vi "runScript.vi"(6 "timeStamp":string, 8 "error in (no error)":errorcluster, 9 "Path":path, 10 "CompiledScript":T1, 11 "BECHWCBasic in":refnum<class "BECHWCBasic.lvclass">) -> (0 "error out":errorcluster, 3 "BECHWCBasic out":refnum<class "BECHWCBasic.lvclass">)   [LabVIEW 2011, in "Hardware.lvlib" / "HWControllers.lvlib" / "BECHWCBasic.lvclass"]
uses:
  BECHWCBasic.lvclass
  Tools/SettingsProcessors/ScriptListCompiler/ScriptListCompiler.lvclass
  Channels/VoltOutput/AnalogOutput.lvclass
  Channels/Digital/DigitalOutput.lvclass
  Channels/DDSOutput/Generic/DDSOutput.lvclass
  HWController.lvclass
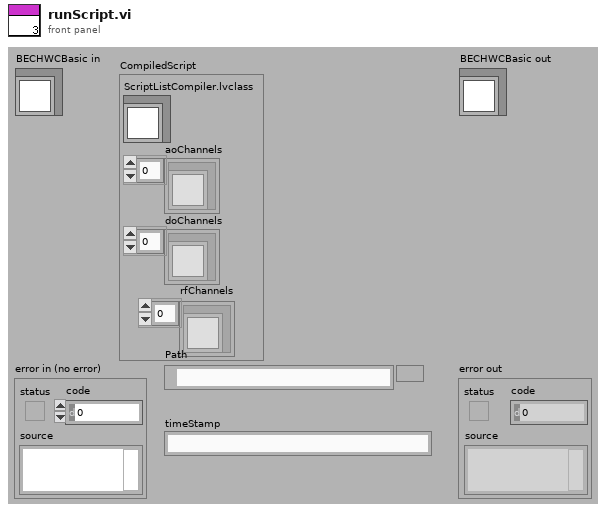
[diagram p1: front panel]
types:
  T1 = cluster{"ScriptListCompiler.lvclass":refnum<class "ScriptListCompiler.lvclass">, "aoChannels":refnum<class "AnalogOutput.lvclass">[], "doChannels":refnum<class "DigitalOutput.lvclass">[], "rfChannels":refnum<class "DDSOutput.lvclass">[]}
  T2 = enum16{"Ready", "Compiling", "Configured", "Running", "Stopping", "Unresolved Error"}
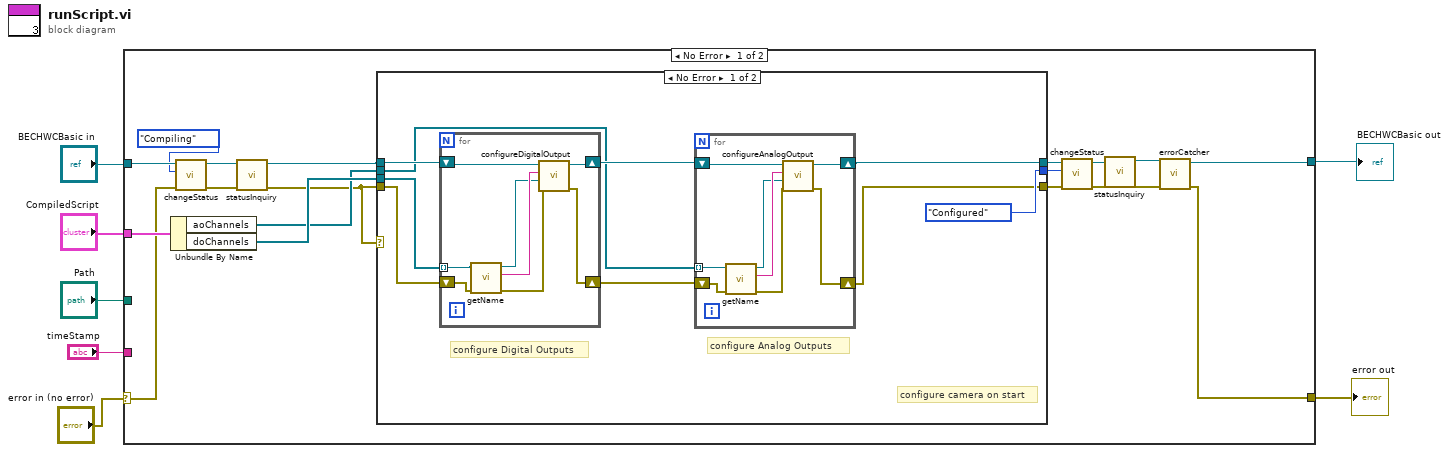
[diagram p0: block diagram]
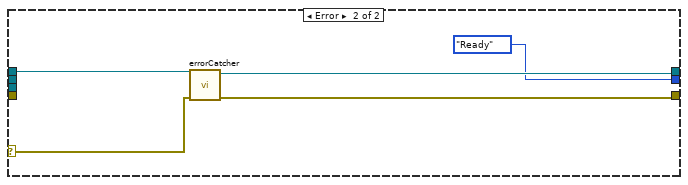
[diagram p2: hidden frame]
diagram:
  n1 = case shown="No Error" "error in (no error)" {
    selector: "error in (no error)" -> [w12 w57]
    tunnel: "BECHWCBasic in" -> [w20 w58]
    tunnel: [w9 w58] -> w5
    tunnel: [w8 w57] -> w4
    tunnel: "CompiledScript" -> [w17 _]
    tunnel: "timeStamp" -> [_ _]
    tunnel: "Path" -> [_ _]
    frame No Error {
      n2 = Unbundle By Name(w17) -> ("aoChannels"=w15:refnum<class "AnalogOutput.lvclass">[], "doChannels"=w16:refnum<class "DigitalOutput.lvclass">[])
      n3 = call "changeStatus.vi"("error in (no error)"=w12, "status"=T2."Compiling", "HWController in"=w20) -> ("error out"=w22:errorcluster, "HWController out"=w21:refnum<class "BECHWCBasic.lvclass">)  [unwired: 7 in]
      n4 = call-dynamic "statusInquiry.vi"("error in (no error)"=w22, "HWController in"=w21) -> ("error out"=w13:errorcluster, "HWController out"=w14:refnum<class "BECHWCBasic.lvclass">)  [unwired: 8 in]
      n5 = case shown="No Error" w13 {
        selector: w13 -> [_ w53]
        tunnel: [w28 w55] -> w26
        tunnel: [w27 w54] -> w25
        tunnel: w14 -> [w34 w56]
        tunnel: w13 -> [w33 _]
        tunnel: w16 -> [w31 _]
        tunnel: w15 -> [w30 _]
        tunnel: [T2."Configured" ("status") T2."Ready" ("status")] -> w18
        frame No Error {
          # "configure camera on start"
          # "configure Analog Outputs"
          # "configure Digital Outputs"
          n6 = for {
            shift-right: [w45] -> w32
            shift-left: w33 -> [w51]
            shift-right: [w49] -> w35
            shift-left: w34 -> [w50]
            tunnel: w31 -> [w44] mode=indexing
            n7 = call-dynamic "getName.vi"("error in (no error)"=w51, "DigitalOutput.lvclass in"=w44) -> ("error out"=w47:errorcluster, "name"=w48:string, "DigitalOutput.lvclass out"=w46:refnum<class "DigitalOutput.lvclass">)  [unwired: 7 in]
            n8 = call "configureDigitalOutput.vi"("error in (no error)"=w47, "DigitalOutput"=w46, "deviceName"=w48, "BECHWCBasic in"=w50) -> ("error out"=w45:errorcluster, "BECHWCBasic out"=w49:refnum<class "BECHWCBasic.lvclass">)  [unwired: 6 in]
          }
          n9 = for {
            tunnel: w30 -> [w36] mode=indexing
            shift-right: [w40] -> w27
            shift-left: w32 -> [w43]
            shift-right: [w41] -> w28
            shift-left: w35 -> [w42]
            n10 = call "getName.vi"("error in (no error)"=w43, "AnalogOutput.lvclass in"=w36) -> ("error out"=w39:errorcluster, "name"=w38:string, "AnalogOutput.lvclass out"=w37:refnum<class "AnalogOutput.lvclass">)  [unwired: 7 in]
            n11 = call "configureAnalogOutput.vi"("error in (no error)"=w39, "AnalogOutput"=w37, "deviceName"=w38, "BECHWCBasic in"=w42) -> ("error out"=w40:errorcluster, "BECHWCBasic out"=w41:refnum<class "BECHWCBasic.lvclass">)  [unwired: 6 in]
          }
        }
        frame Error {
          n12 = call-dynamic "errorCatcher.vi"("error in (no error)"=w53, "HWController in"=w56) -> ("error out"=w54:errorcluster, "HWController out"=w55:refnum<class "BECHWCBasic.lvclass">)  [unwired: 8 in]
        }
      }
      n13 = call "changeStatus.vi"("error in (no error)"=w25, "status"=w18, "HWController in"=w26) -> ("error out"=w24:errorcluster, "HWController out"=w23:refnum<class "BECHWCBasic.lvclass">)  [unwired: 7 in]
      n14 = call-dynamic "statusInquiry.vi"("error in (no error)"=w24, "HWController in"=w23) -> ("error out"=w10:errorcluster, "HWController out"=w11:refnum<class "BECHWCBasic.lvclass">)  [unwired: 8 in]
      n15 = call-dynamic "errorCatcher.vi"("error in (no error)"=w10, "HWController in"=w11) -> ("error out"=w8:errorcluster, "HWController out"=w9:refnum<class "BECHWCBasic.lvclass">)  [unwired: 8 in]
    }
    frame Error {
    }
  }
  "error out" <- w4
  "BECHWCBasic out" <- w5
